vi "global.vi"() -> ()   [LabVIEW 2015]
panel:
  out "pc2 output":string
  out "pc1 output":string
  in  "stop":bool
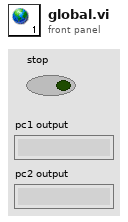
[diagram p1: front panel]
diagram:
